vi "Destroy WyPt Dict.vi"(8 "error in (no error)":errorcluster) -> (0 "error out":errorcluster)   [LabVIEW 2020, in "WyPtDict.lvlib"]
uses:
  WyPtDict.lvlib
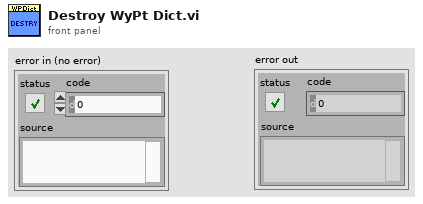
[diagram p1: front panel]
types:
  T1 = typedef "TD Dynamic CVT DVR--ref.ctl" = refnum<data-value>
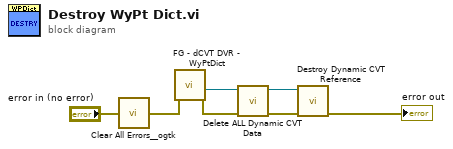
[diagram p0: block diagram]
diagram:
  n1 = call <userlib>:"Clear All Errors__ogtk.vi"("Error In"="error in (no error)") -> ("Error Out"=w1:errorcluster)  [unwired: 3 in]
  n2 = call "FG - dCVT DVR - WyPtDict.vi"("error in (no error)"=w1) -> ("dCVT WyPt out"=w5:T1, "error out"=w3:errorcluster)  [unwired: 8 in]
  n3 = call <vilib>:"Delete ALL Dynamic CVT Data.vi"("error in (no error)"=w3, "dCVT DVR"=w5) -> ("error out"=w6:errorcluster, "dCVT DVR out"=w2:T1)  [unwired: 8 in]
  n4 = call <vilib>:"Destroy Dynamic CVT Reference.vi"("error in (no error)"=w6, "dCVT DVR"=w2) -> ("error out"=→"error out":errorcluster)  [unwired: 8 in, 1 out]
